vi "Initial Bearing.vi"(0 "Latitude":dbl, 1 "North or South":string, 2 "Longitude":dbl, 3 "East or West":string, 4 "Destination Latitude":dbl, 5 "Destination N/S":string, 6 "Destination Longitude":dbl, 7 "Destination E/W":string) -> (20 "Initial Bearing":dbl(xcontrol))   [LabVIEW 2011]
uses:
  <vilib>/robotics/Controls/Compass Indicator/Compass Indicator.xctl
  <vilib>/express/express arith-compare/Formula/XNode/ExpressFormulaBlockNode.xnode
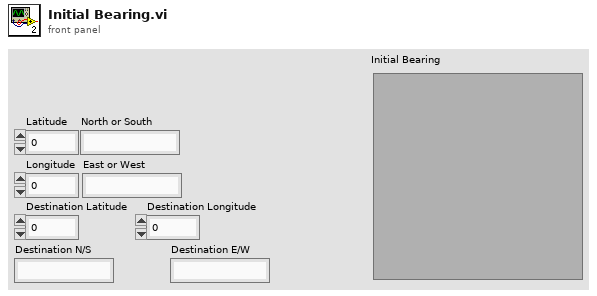
[diagram p1: front panel]
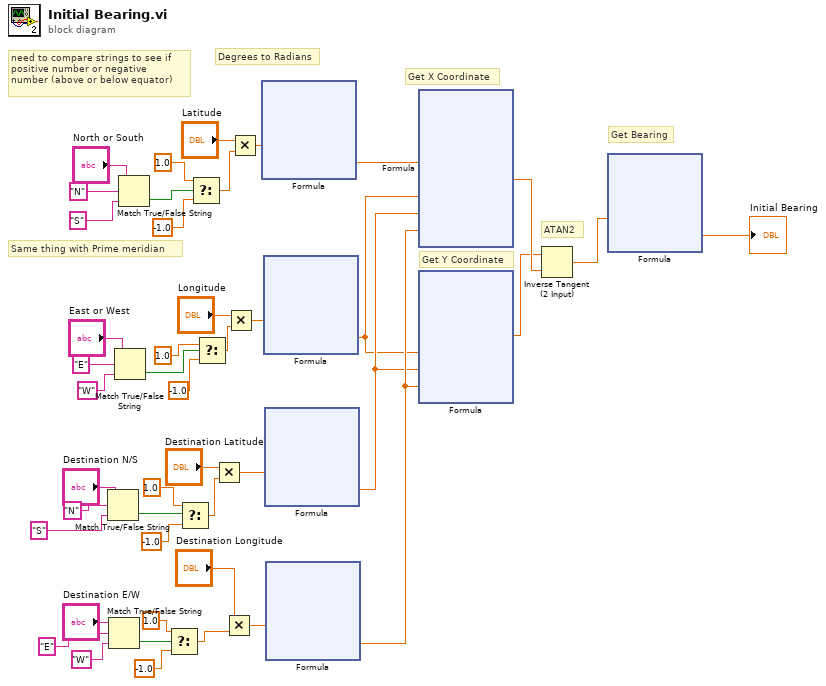
[diagram p0: block diagram]
diagram:
  # "Same thing with Prime meridian"
  # "need to compare strings to see if \npositive number or negative \nnumber (above or below equator)"
  # "Get Bearing"
  # "ATAN2"
  # "Get Y Coordinate"
  # "Get X Coordinate"
  # "Degrees to Radians"
  n1 = Match True/False String(2:"S" ("false string"), 3:"N" ("true string"), 4:"Destination N/S") -> (0:w41:bool)  [unwired: 1 out]
  n2 = Match True/False String(2:"W" ("false string"), 3:"E" ("true string"), 4:"Destination E/W") -> (0:w33:bool)  [unwired: 1 out]
  n3 = Match True/False String(2:"W" ("false string"), 3:"E" ("true string"), 4:"East or West") -> (0:w24:bool)  [unwired: 1 out]
  n4 = Match True/False String(2:"S" ("false string"), 3:"N" ("true string"), 4:"North or South") -> (0:w21:bool)  [unwired: 1 out]
  n5 = Select(t=1.0, s=w33, f=-1.0) -> (s? t:f=w43:dbl)
  n6 = Select(t=1.0, s=w41, f=-1.0) -> (s? t:f=w42:dbl)
  n7 = Select(t=1.0, s=w21, f=-1.0) -> (s? t:f=w28:dbl)
  n8 = Select(t=1.0, s=w24, f=-1.0) -> (s? t:f=w27:dbl)
  n9 = Multiply(x="Destination Latitude", y=w42) -> (x*y=w32:dbl)
  n10 = Multiply(x="Destination Longitude", y=w43) -> (x*y=w31:dbl)
  n11 = Multiply(x="Longitude", y=w27) -> (x*y=w29:dbl)
  n12 = Multiply(x="Latitude", y=w28) -> (x*y=w30:dbl)
  n13 = xnode "Formula"("Dlat1"=w30) -> ("Result"=w10:dbl)  [unwired: 1 in, 1 out]
  n14 = xnode "Formula"("Dlong1"=w29) -> ("Result"=w9:dbl)  [unwired: 1 in, 1 out]
  n15 = xnode "Formula"("Dlat2"=w32) -> ("Result"=w12:dbl)  [unwired: 1 in, 1 out]
  n16 = xnode "Formula"("Dlong2"=w31) -> ("Result"=w13:dbl)  [unwired: 1 in, 1 out]
  n17 = xnode "Formula"("CurLat"=w10, "CurLong"=w9, "DesLat"=w12, "DesLong"=w13) -> ("Result"=w15:dbl)  [unwired: 1 in, 1 out]
  n18 = xnode "Formula"("CurLong"=w9, "DesLat"=w12, "DesLong"=w13) -> ("Result"=w14:dbl)  [unwired: 1 in, 1 out]
  n19 = Inverse Tangent (2 Input)(1:w15, 2:w14) -> (0:w16:dbl)
  n20 = xnode "Formula"("rad"=w16) -> ("Result"=→"Initial Bearing":dbl)  [unwired: 1 in, 1 out]
